vi "Engine - Generic - Specifications Host.vi"() -> ()   [LabVIEW 2015, in "ECS-Host.lvlib"]
uses:
  ECS-Host.lvlib
panel:
  in  "Q.LHV Fuel":sgl caption="[]"
  in  "StoichAFR":sgl caption="[]"
  in  "NumberOfCyl":u8
  in  "EngineDisplacement":sgl caption="[]"
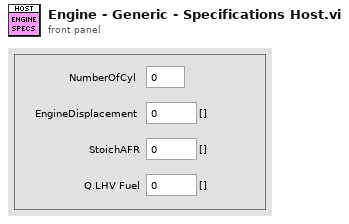
[diagram p1: front panel]
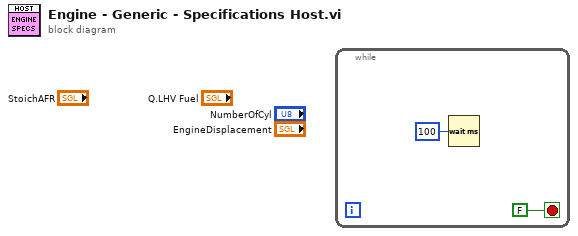
[diagram p0: block diagram]
diagram:
  n1 = while {
    stop <- FALSE stop-if-true
    n2 = Wait (ms)(milliseconds to wait=u32 100) -> ()  [unwired: 1 out]
  }
